vi "Exercise 10.4.vi"() -> ()   [LabVIEW 2020]
panel:
  out "Locked/Unlocked":bool
  in  "Clear":bool
  out "Code Entered":string
  in  "Enter":bool
  in  "Button 9":bool
  in  "Button 8":bool
  in  "Button 7":bool
  in  "Button 6":bool
  in  "Button 5":bool
  in  "Button 4":bool
  in  "Button 3":bool
  in  "Button 2":bool
  in  "Button 1":bool
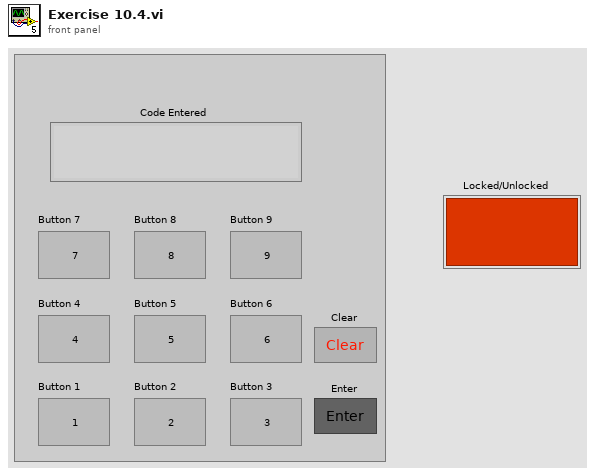
[diagram p1: front panel]
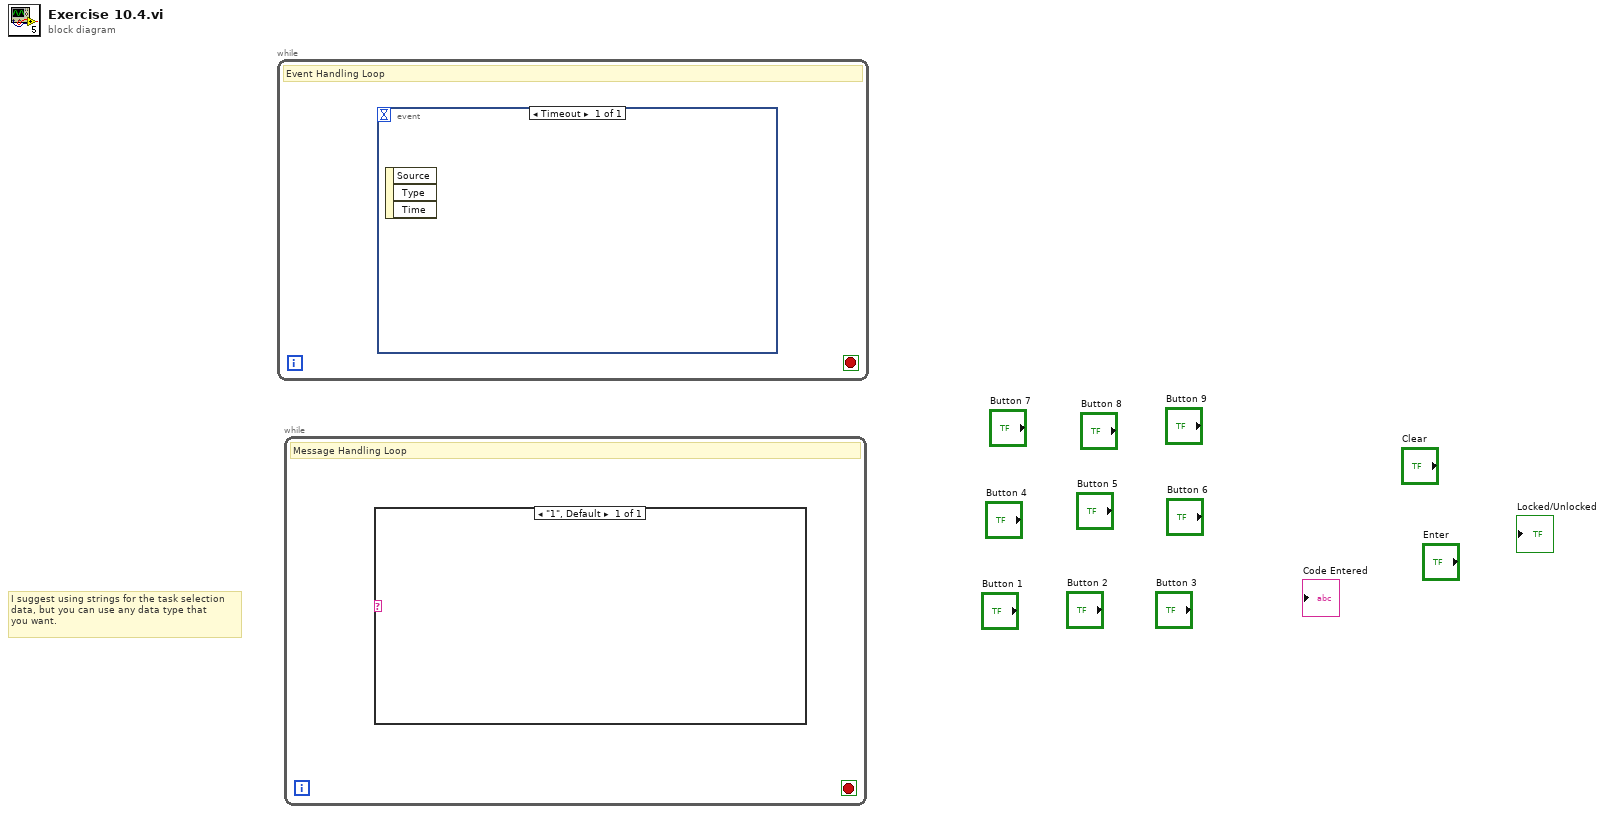
[diagram p0: block diagram]
diagram:
  # "I suggest using strings for the task selection\ndata, but you can use any data type that\nyou want."
  n1 = while {
    stop <- _ stop-if-true
    # "Event Handling Loop"
    n2 = event shown="[0] Timeout" {
      selector: _ -> [_]
      dyn-events: _ -> [_]
      timeout: _ -> [_]
      event Timeout {
        n3 = event-data() -> ()  [unwired: 1 in, 3 out]
      }
    }
  }
  n4 = while {
    stop <- _ stop-if-true
    # "Message Handling Loop"
    n5 = case shown="\"1\", Default" {
      selector: _ -> [_]
      frame "1", Default {
      }
    }
  }
